vi "GEM_BANK_ARRAY_BuildHeader.vi"(2 "BANK NUMBER":u32, 3 "Number of LVBANK entries":i32, 4 "Size of data bundle":u32) -> (0 "output":u8[](array[numeric]))   [LabVIEW 2018, in "GEM_BANK_ARRAY.lvclass"]
uses:
  GEM_BANK_ARRAY.lvclass
panel:
  out "resulting string (Plan text)":string
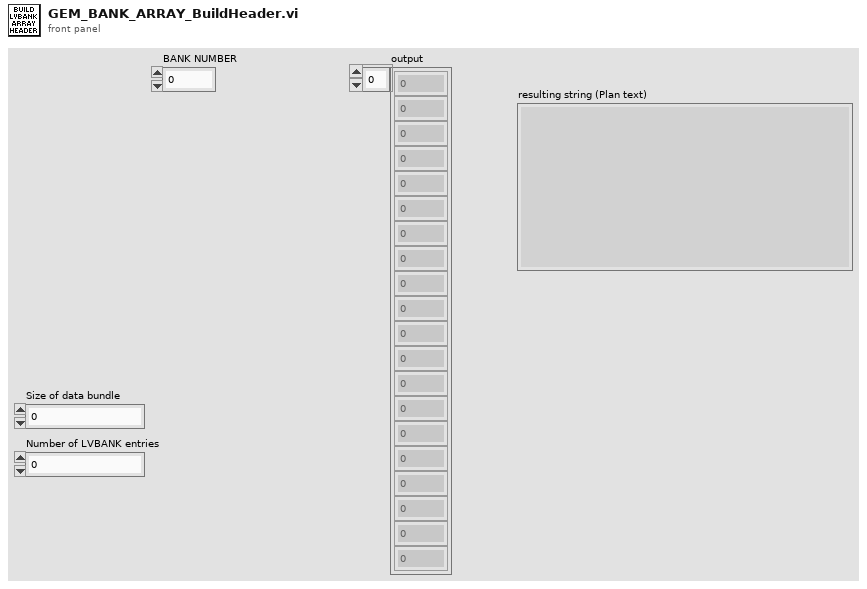
[diagram p1: front panel]
types:
  T1 = enum16{"big-endian, network order", "native, host order", "little-endian"}
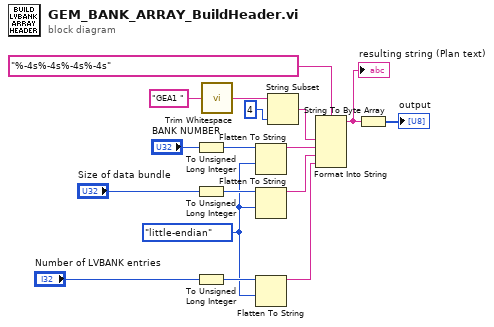
[diagram p0: block diagram]
diagram:
  w3 = T1."little-endian" ("byte order (0:big-endian, network order)")
  n1 = To Unsigned Long Integer(number="BANK NUMBER") -> (unsigned 32bit integer=w4:u32)
  n2 = To Unsigned Long Integer(number="Size of data bundle") -> (unsigned 32bit integer=w15:u32)
  n3 = To Unsigned Long Integer(number="Number of LVBANK entries") -> (unsigned 32bit integer=w14:u32)
  n4 = call <vilib>:"Trim Whitespace.vi"("string"="GEA1 ") -> ("trimmed string"=w12:string)  [unwired: 1 in]
  n5 = Flatten To String(anything=w4, byte order (0:big-endian, network order)=w3) -> (data string=w2:string)  [unwired: 2 in, 2 out]
  n6 = Flatten To String(anything=w15, byte order (0:big-endian, network order)=w3) -> (data string=w5:string)  [unwired: 2 in, 2 out]
  n7 = Flatten To String(anything=w14, byte order (0:big-endian, network order)=w3) -> (data string=w6:string)  [unwired: 2 in, 2 out]
  n8 = String Subset(string=w12, length (rest)=4 ("length (rest)")) -> (substring=w11:string)  [unwired: 1 in]
  n9 = Format Into String(format string="%-4s%-4s%-4s%-4s", w11, w2, w5, w6) -> (resulting string=w8:string)  [unwired: 2 in, 1 out]
  "resulting string (Plan text)" <- w8
  n10 = String To Byte Array(string=w8) -> (unsigned byte array=→"output":u8[])
